vi "NONBLOCKING_TIMER.vi"(2 "Start on Value Changed":bool, 3 "Time to Wait":dbl) -> (0 "Elapsed Time":dbl format="%#_13g", 1 "Timer Has Elapsed":bool)   [LabVIEW 2013]
doc: "Really just a wrapper for the Elapsed Time express subvi, with some trigger functionality built in so that the timer resets when the input (e.g. state) changes."
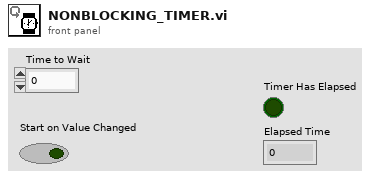
[diagram p1: front panel]
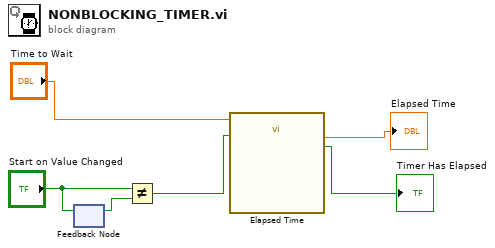
[diagram p0: block diagram]
diagram:
  n1 = feedback-in #1("Start on Value Changed") -> ()
  n2 = feedback #1() -> (w1:bool)  [unwired: 1 in]
  n3 = Not Equal?(x="Start on Value Changed", y=w1) -> (x != y?=w3:bool)
  n4 = call "Elapsed Time"("Time Target (s)"="Time to Wait", "Reset"=w3) -> ("Elapsed Time (s)"=→"Elapsed Time":dbl, "Time has Elapsed"=→"Timer Has Elapsed":bool)  [unwired: 10 in, 6 out]
